vi "CLIENT-TCP-IP.vi"(10 "SERVER IP address":string(combo)="localhost") -> ()   [LabVIEW 2015]
uses:
  <vilib>/NI/STM/NI STM.lvlib
  <vilib>/NI/STM/TCP/Read Message (TCP).vi
  <vilib>/NI/STM/TCP/Write Message (TCP).vi
  Clusters-def/SERVER-Commands.ctl
  <vilib>/NI/STM/TCP/Read Meta Data (TCP Ref).vi
panel:
  in  "Channel":i32 min=0 max=3 step=1
  in  "Stop Host":bool
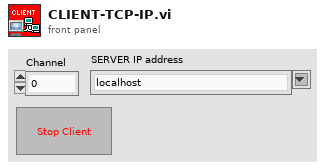
[diagram p1: front panel]
types:
  T1 = typedef "NI STM.lvlib/TCP Connection Info.ctl" = cluster{"connection ID":refnum<k5>, "meta data":T2[]}
  T2 = typedef "NI STM.lvlib/MetaDataElement.ctl" = string
  T3 = typedef "SERVER-Commands.ctl" = string
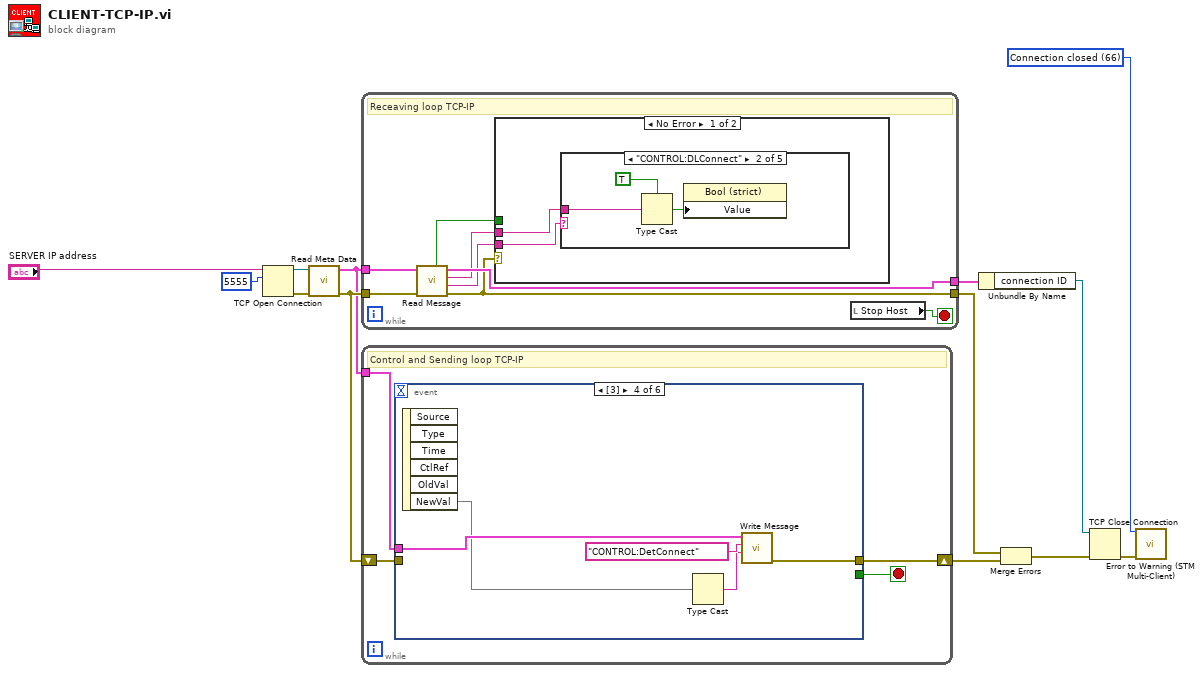
[diagram p0: block diagram]
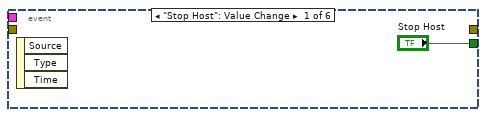
[diagram p2: hidden frame]
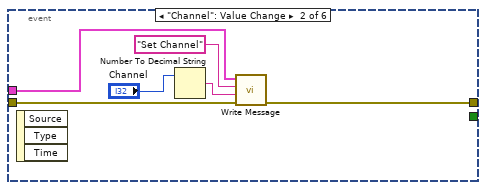
[diagram p3: hidden frame]
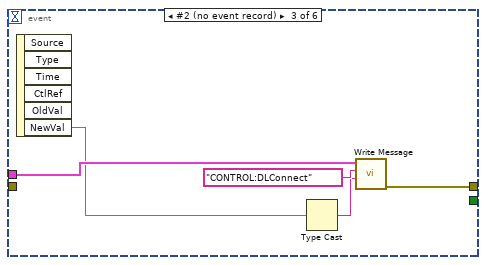
[diagram p4: hidden frame]
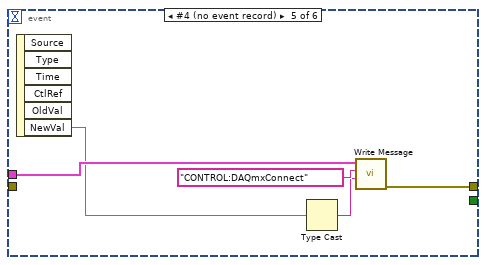
[diagram p5: hidden frame]
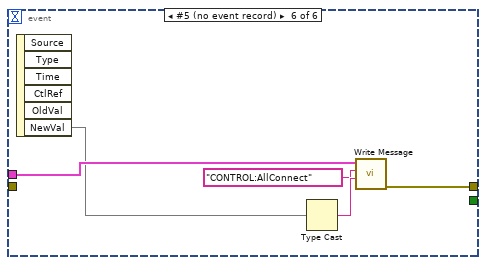
[diagram p6: hidden frame]
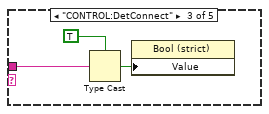
[diagram p8: hidden frame]
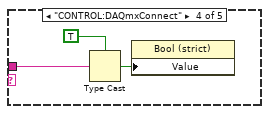
[diagram p9: hidden frame]
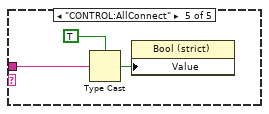
[diagram p10: hidden frame]
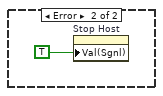
[diagram p11: hidden frame]
diagram:
  w7 = 66 items=["No Error", "Argument Error", "Memory Full", "Out of Zone", "End of File", "File Already Open", "Generic File IO Error", "File Not Found", "File Permission Error", "Disk Full", "Duplicate Path", "Too Many Files Open", "Not Enabled", "Resource File Not Found", "Cannot Add Resource", "Resource Not Found", "Image Not Found", "Image Memory Error", "Pen Does Not Exist", "Config Bad Type", "Config Token Not Found", "Config Parse Error", "Config Memory Error", "Bad External Code Format", "Bad External Code Offset", "External Code Not Present", "Null Window", "Destroy Window Mixup", "Null Menu", "Print Aborted", "Bad Print Record", "Print Driver Error", "Windows Error During Print", "Memory Error During Print", "Print Dialog Error", "Generic Print Error", "Invalid Device Refnum", "Device Not Found", "Device Parameter Error", "Device Unit Error", "Can't Open Device", "Device Call Aborted", "Generic Error", "Cancelled By User", "Object ID Too Low", "Object ID Too High", "Object Not In Heap", "Unknown Heap", "Bad DefProc ID", "DefProc Not In Table", "Message Out Of Range", "Null Method", "Unknown Message", "Manager Call Not Supported", "Bad address", "Connection In progress", "Connection timed out", "Connection is already in progress", "Network attribute not supported", "Network error", "Address in use", "System out of memory", "Connection aborted", "Connection refused", "Connection is not connected", "Connection is already connected", "Connection closed", "Initialize error (interapplication manager)", "Bad occurrence", "Wait on unbound occurrence handler", "Occurrence queue overflow", "Bad path", "Semaphore not signaled", "Unrecognized type (interapplication manager)"] ("1st Error to Convert")
  n1 = TCP Open Connection(address="SERVER IP address", remote port or service name=u16 5555 ("remote port")) -> (connection ID=w2:refnum<k5>, error out=w3:errorcluster)  [unwired: 3 in]
  n2 = call-poly <vilib>:"Read Meta Data.vi"("error in"=w3, "connection ID"=w2) -> ("error out"=w12:errorcluster, "connection info out"=w5:T1)  [unwired: 7 in, 1 out]
  n3 = while {
    tunnel: w5 -> [w14]
    tunnel: w12 -> [w21]
    tunnel: [w20] -> w11
    tunnel: [w15] -> w9
    stop <- w16 stop-if-true
    # "Receaving loop TCP-IP"
    n4 = call-poly <vilib>:"Read Message.vi"("error in"=w21, "connection info in"=w14) -> ("error out"=w15:errorcluster, "name"=w19:T2, "data string"=w18:string, "connection info out"=w20:T1, "timed out?"=w17:bool)  [unwired: 4 in, 1 out]
    n5 = case shown="No Error" w15 {
      tunnel: w19 -> [w23 _]
      tunnel: w18 -> [w22 _]
      tunnel: w17 -> [_ _]
      frame No Error {
        n6 = case shown="\"CONTROL:DLConnect\"" w23 {
          tunnel: w22 -> [_ w25 w28 w31 w34]
          frame Default {
          }
          frame "CONTROL:DLConnect" {
            n7 = Type Cast(type=TRUE, x=w25) -> (*(type *) &x=w24:bool)
            n8 = property on="Property Node" class="Bool (strict)"("Value"=w24) -> ()  [unwired: 2 in, 2 out]
          }
          frame "CONTROL:DetConnect" {
            n9 = Type Cast(type=TRUE, x=w28) -> (*(type *) &x=w27:bool)
            n10 = property on="Property Node" class="Bool (strict)"("Value"=w27) -> ()  [unwired: 2 in, 2 out]
          }
          frame "CONTROL:DAQmxConnect" {
            n11 = Type Cast(type=TRUE, x=w31) -> (*(type *) &x=w30:bool)
            n12 = property on="Property Node" class="Bool (strict)"("Value"=w30) -> ()  [unwired: 2 in, 2 out]
          }
          frame "CONTROL:AllConnect" {
            n13 = Type Cast(type=TRUE, x=w34) -> (*(type *) &x=w33:bool)
            n14 = property on="Property Node" class="Bool (strict)"("Value"=w33) -> ()  [unwired: 2 in, 2 out]
          }
        }
      }
      frame Error {
        n15 = property on="Stop Host" class="Bool (strict)"("Val(Sgnl)"=TRUE ("Value (Signaling)")) -> ()  [unwired: 2 in, 2 out]
      }
    }
    n16 = local read "Stop Host"() -> (w16:bool)
  }
  n17 = while {
    tunnel: w5 -> [w40]
    shift-right: [w37] -> w10
    shift-left: w12 -> [w39]
    stop <- w38 stop-if-true
    # "Control and Sending loop TCP-IP"
    n18 = event shown="[3]" {
      selector: _ -> [_ _ _ _ _ _]
      dyn-events: _ -> [_ _ _ _ _ _]
      timeout: _ -> [_ _ _ _ _ _]
      tunnel: w40 -> [_ w43 w51 w56 w61 w66]
      tunnel: w39 -> [_ w45 _ _ _ _]
      tunnel: ["Stop Host" _ _ _ _ _] -> w38
      tunnel: [_ w44 w52 w57 w62 w67] -> w37
      event "Stop Host": Value Change {
        n19 = event-data() -> ()  [unwired: 1 in, 3 out]
      }
      event "Channel": Value Change {
        n20 = event-data() -> ()  [unwired: 1 in, 3 out]
        n21 = Number To Decimal String(number="Channel") -> (decimal integer string=w46:string)  [unwired: 1 in]
        n22 = call-poly <vilib>:"Write Message.vi"("error in"=w45, "data"=w46, "name"="Set Channel" ("Name"), "connection info in"=w43) -> ("error out"=w44:errorcluster)  [unwired: 6 in, 1 out]
      }
      event #2 (no event record) {
        n23 = event-data() -> ("NewVal"=w49)  [unwired: 1 in, 5 out]
        n24 = Type Cast(x=w49) -> (*(type *) &x=w48:string)  [unwired: 1 in]
        n25 = call-poly <vilib>:"Write Message.vi"("data"=w48, "name"=T3 "CONTROL:DLConnect" ("Commands"), "connection info in"=w51) -> ("error out"=w52:errorcluster)  [unwired: 7 in, 1 out]
      }
      event #3 (no event record) {
        n26 = event-data() -> ("NewVal"=w54)  [unwired: 1 in, 5 out]
        n27 = Type Cast(x=w54) -> (*(type *) &x=w53:string)  [unwired: 1 in]
        n28 = call-poly <vilib>:"Write Message.vi"("data"=w53, "name"=T3 "CONTROL:DetConnect" ("Commands"), "connection info in"=w56) -> ("error out"=w57:errorcluster)  [unwired: 7 in, 1 out]
      }
      event #4 (no event record) {
        n29 = event-data() -> ("NewVal"=w59)  [unwired: 1 in, 5 out]
        n30 = Type Cast(x=w59) -> (*(type *) &x=w58:string)  [unwired: 1 in]
        n31 = call-poly <vilib>:"Write Message.vi"("data"=w58, "name"=T3 "CONTROL:DAQmxConnect" ("Commands"), "connection info in"=w61) -> ("error out"=w62:errorcluster)  [unwired: 7 in, 1 out]
      }
      event #5 (no event record) {
        n32 = event-data() -> ("NewVal"=w65)  [unwired: 1 in, 5 out]
        n33 = Type Cast(x=w65) -> (*(type *) &x=w64:string)  [unwired: 1 in]
        n34 = call-poly <vilib>:"Write Message.vi"("data"=w64, "name"=T3 "CONTROL:AllConnect" ("Commands"), "connection info in"=w66) -> ("error out"=w67:errorcluster)  [unwired: 7 in, 1 out]
      }
    }
  }
  n35 = Unbundle By Name(w11) -> ("connection ID"=w13:refnum<k5>)
  n36 = Merge Errors(w9, w10) -> (w8:errorcluster)
  n37 = TCP Close Connection(connection ID=w13, error in (no error)=w8) -> (error out=w6:errorcluster)  [unwired: 1 in, 1 out]
  n38 = call "Error to Warning (STM Multi-Client).vi"("1st Error to Convert"=w7, "error in"=w6) -> ()  [unwired: 13 in, 1 out]
